vi "KTable Test.vi"() -> ()   [LabVIEW 2015]
uses:
  KTable/KTable.xctl
panel:
  in  "Palette":bool
  out "event":string
  in  "Default":T1={"Val1"="Sucks", "Val2"=96, "Boolean"=TRUE, "Val3"=5, "formula"="x = y^2"}
  out "data":T2(array[cluster])
  in  "Array":T3(array[cluster])=[{"Val1"="argh", "Val2"=0.0, "Boolean"=TRUE, "Val3"=0, "formula"=""}, {"Val1"="Shit", "Val2"=15.0, "Boolean"=FALSE, "Val3"=1, "formula"="x = y^2"}, {"Val1"="Dafuq", "Val2"=3.0, "Boolean"=TRUE, "Val3"=0, "formula"="x = y^3"}]
  in  "stop":bool
  in  "KTable":u16(xcontrol)
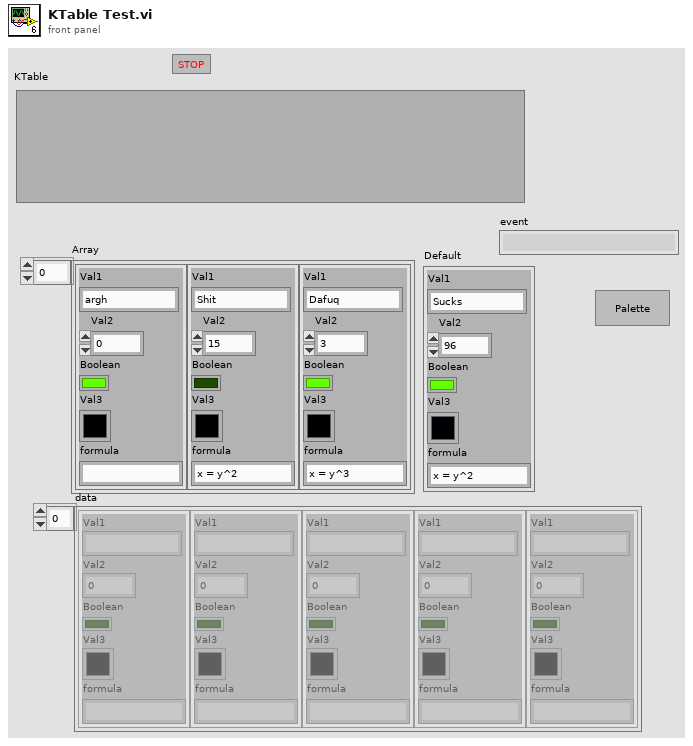
[diagram p1: front panel]
types:
  T1 = cluster{"Val1":string, "Val2":i32, "Boolean":bool, "Val3":u32, "formula":string}
  T2 = cluster{"Val1":string, "Val2":i32, "Boolean":bool, "Val3":u32, "formula":string}[]
  T3 = cluster{"Val1":string, "Val2":dbl, "Boolean":bool, "Val3":u32, "formula":string}[]
  T4 = typedef "KTable.xctl/Events.ctl" = cluster{"Items Changed":refnum<user-event>}
  T5 = typedef "KTable.xctl/Event Type.ctl" = enum16{"None", "Selection", "Edit", "Insert", "Delete", "Up", "Down", "Duplicate"}
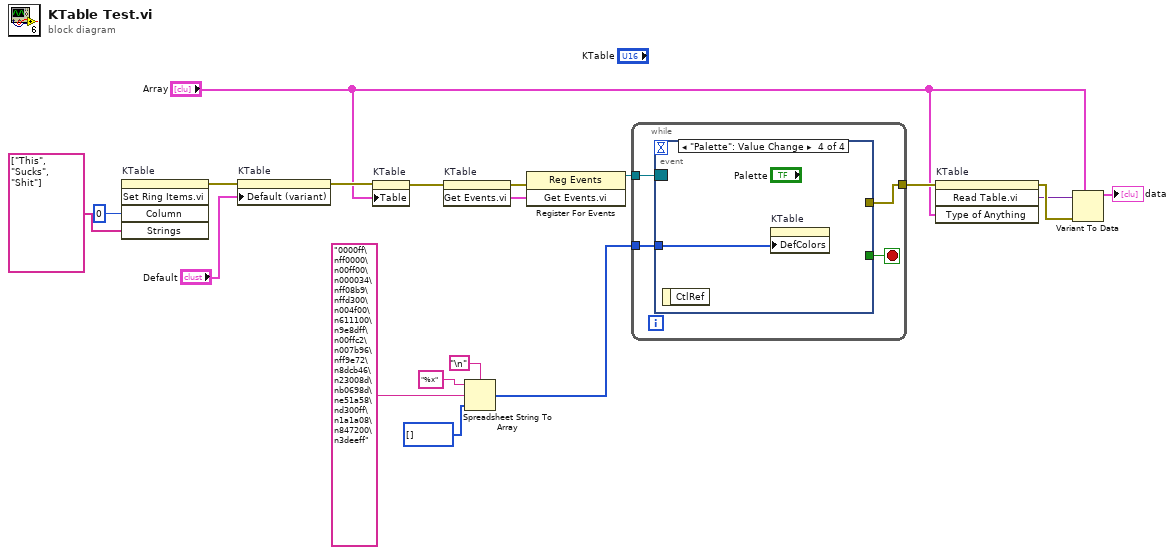
[diagram p0: block diagram]
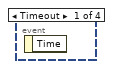
[diagram p2: hidden frame]
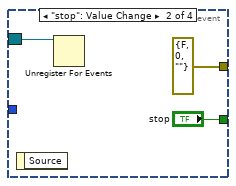
[diagram p3: hidden frame]
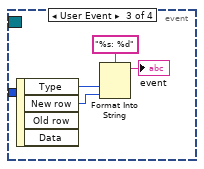
[diagram p4: hidden frame]
diagram:
  n1 = invoke on="KTable" class="KTable (strict)" method="Set Ring Items.vi"("Column"=0, "Strings"=string[] ["This", "Sucks", "Shit"]) -> (error out=w15:errorcluster)  [unwired: 3 in, 4 out]
  n2 = property on="KTable" class="KTable (strict)"(error in=w15, "Default (variant)"="Default") -> (error out=w14:errorcluster)  [unwired: 1 in, 1 out]
  n3 = property on="KTable" class="KTable (strict)"(error in=w14, "Table"="Array") -> (error out=w12:errorcluster)  [unwired: 1 in, 1 out]
  n4 = invoke on="KTable" class="KTable (strict)" method="Get Events.vi"(error in=w12) -> (error out=w11:errorcluster, "Get Events.vi"=w10:T4)  [unwired: 2 in, 1 out]
  n5 = Spreadsheet String To Array(delimiter (Tab)="\n", format string="%x", spreadsheet string="0000ff\nff0000\n00ff00\n000034\nff08b9\nffd300\n004f00\n611100\n9e8dff\n00ffc2\n007b96\nff9e72\n8dcb46\n23008d\nb0698d\ne51a58\nd300ff\n1a1a08\n847200\n3deeff", array type (2D Dbl)=u32[] []) -> (array=w2:u32[])
  n6 = register-events(error in=w11, w10) -> (reference out=w7:refnum<event-registration>)  [unwired: 1 in, 1 out]
  n7 = while {
    tunnel: [w22] -> w18
    tunnel: w7 -> [w21]
    tunnel: w2 -> [w20]
    stop <- w23 stop-if-true
    n8 = event shown="[3] \"Palette\": Value Change" {
      selector: w21 -> [_ w25 _ _]
      dyn-events: _ -> [_ _ _ _]
      timeout: _ -> [_ _ _ _]
      tunnel: [_ "stop" _ _] -> w23
      tunnel: [_ errorcluster {"status"=FALSE, "code"=0, "source"=""} ("error constant") _ _] -> w22
      tunnel: w20 -> [_ _ _ w31]
      event Timeout {
        n9 = event-data() -> ()  [unwired: 1 in, 1 out]
      }
      event "stop": Value Change {
        n10 = event-data() -> ()  [unwired: 1 in, 1 out]
        n11 = Unregister For Events(event registration refnum=w25) -> ()  [unwired: 1 in, 1 out]
      }
      event User Event {
        n12 = event-data() -> ("Type"=w29:T5, "New row"=w28:i32)  [unwired: 1 in, 2 out]
        n13 = Format Into String(format string="%s: %d", w29, w28) -> (resulting string=→"event":string)  [unwired: 2 in, 1 out]
      }
      event "Palette": Value Change {
        n14 = event-data() -> ()  [unwired: 1 in, 1 out]
        n15 = property on="KTable" class="KTable (strict)"("DefColors"=w31) -> ()  [unwired: 2 in, 2 out]
      }
    }
  }
  n16 = invoke on="KTable" class="KTable (strict)" method="Read Table.vi"(error in=w18, "Type of Anything"="Array") -> (error out=w17:errorcluster, "Read Table.vi"=w16:variant)  [unwired: 2 in, 2 out]
  n17 = Variant To Data(error in=w17, type="Array", Variant=w16) -> (data=→"data":T3)  [unwired: 1 out]
